vi "TCL Get Fragments - NeventNfrag.vi"(0 "event file":path, 1 "event numbers":i32[](array[numeric]), 3 "primary key":string, 4 "fragments":string[](array[string]), 5 "error in (no error)":errorcluster) -> (6 "fragments out":string[](array[string]), 7 "values":string[][](array[string]), 8 "error out":errorcluster)   [LabVIEW 2010]
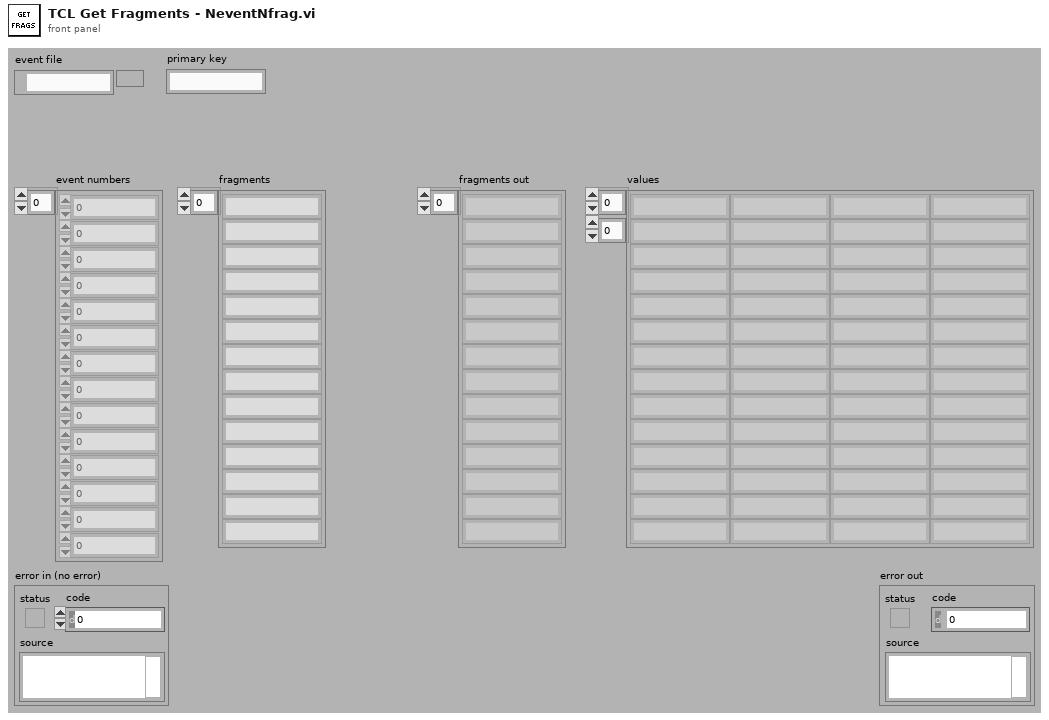
[diagram p1: front panel]
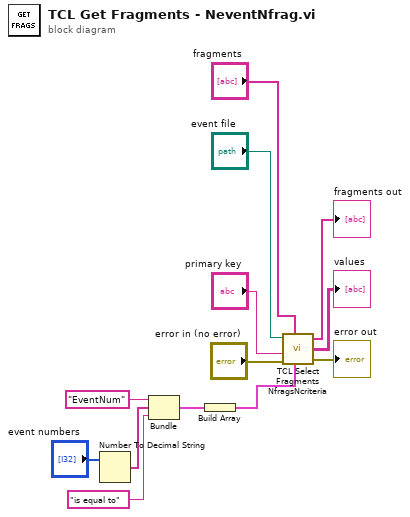
[diagram p0: block diagram]
diagram:
  n1 = Number To Decimal String(number="event numbers") -> (decimal integer string=w6:string[])  [unwired: 1 in]
  n2 = Bundle("EventNum", w6, "is equal to") -> (w10:cluster{string, string[], string})  [unwired: 1 in]
  n3 = Build Array(w10) -> (w8:cluster{string, string[], string}[])
  n4 = call "TCL Select Fragments NfragsNcriteria.vi"("event file"="event file", "fragments"="fragments", "primary key"="primary key", "criteria"=w8, "error in (no error)"="error in (no error)") -> ("fragments out"=→"fragments out":string[], "matches"=→"values":string[][], "error out"=→"error out":errorcluster)  [unwired: 1 in]
